vi "Commit for SET (Remove this later).vi"(0 "Session Handle in":T1, 11 "error in (no error)":errorcluster) -> (4 "Session Handle out":T1, 15 "error out":errorcluster)   [LabVIEW 2015, in "SLSC Switch.lvlib" / "SLSC Session.lvclass"]
uses:
  SLSC Session.lvclass
  Typedefs/Session Handle.ctl
  SLSC Session.lvclass/SLSC Session.ctl
  <vilib>/SLSC/Execute Phys Chan Command.vi
  <vilib>/SLSC/Execute Device Command.vi
  <vilib>/SLSC/SLSC.lvlib
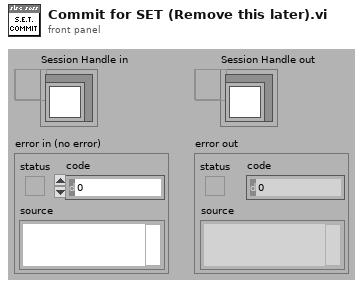
[diagram p1: front panel]
types:
  T1 = typedef "SLSC Switch.lvlib/SLSC Session.lvclass/Session Handle.ctl" = refnum<data-value>
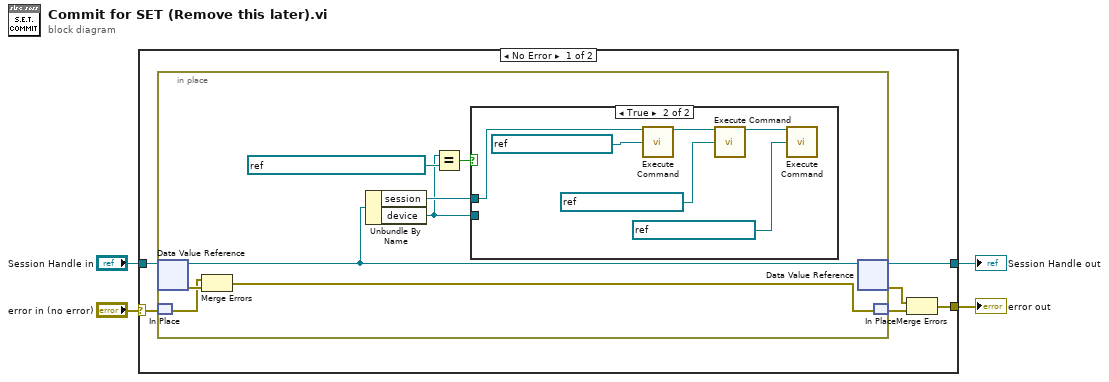
[diagram p0: block diagram]
diagram:
  n1 = case shown="No Error" "error in (no error)" {
    selector: "error in (no error)" -> [w5 w25]
    tunnel: "Session Handle in" -> [w10 w26]
    tunnel: [w9 w26] -> w3
    tunnel: [w6 w25] -> w2
    frame No Error {
      n2 = in-place {
        n3 = in-place-dvr #1(w10) -> (w15:refnum<class "SLSC Session.lvclass">, w17:errorcluster)
        n4 = in-place-match #2(w5) -> (w16:errorcluster)
        n5 = Merge Errors(w16, w17) -> (w18:errorcluster)
        n6 = Unbundle By Name(w15) -> ("session"=w14:refnum<k21>, "device"=w12:refnum<k21>)
        n7 = Equal?(x=w12, y=refnum<k21> "SLSC-12001-030E3F09-Mod6" ("devices")) -> (x = y?=w11:bool)
        n8 = case shown="True" w11 {
          tunnel: w14 -> [_ w24]
          tunnel: w12 -> [_ _]
          frame False {
          }
          frame True {
            n9 = call-poly <vilib>:"Execute Command.vi"("session in"=w24, "command"=refnum<k21> "SET.Base.Commit") -> ("session out"=w23:refnum<k21>)  [unwired: 12 in, 1 out]
            n10 = call-poly <vilib>:"Execute Command.vi"("session in"=w23, "command"=refnum<k21> "SET.Slot1.Commit") -> ("session out"=w22:refnum<k21>)  [unwired: 12 in, 1 out]
            n11 = call-poly <vilib>:"Execute Command.vi"("session in"=w22, "command"=refnum<k21> "SET.Slot2.Commit") -> ()  [unwired: 12 in, 2 out]
          }
        }
        n12 = in-place-dvr #1(w15) -> (w9:T1, w7:errorcluster)
        n13 = in-place-match #2(w18) -> (w8:errorcluster)
      }
      n14 = Merge Errors(w7, w8) -> (w6:errorcluster)
    }
    frame Error {
    }
  }
  "Session Handle out" <- w3
  "error out" <- w2
